vi "REV RPM to ft per s.vi"(11 "Drive Velocities (RPM)":T1) -> (3 "Drive Velocities (ft/s)":T1)   [LabVIEW 2020]
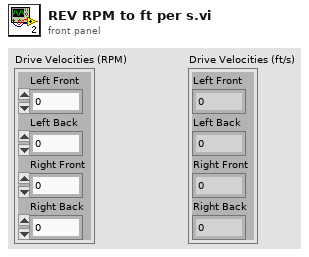
[diagram p1: front panel]
types:
  T1 = cluster{"Left Front":dbl, "Left Back":dbl, "Right Front":dbl, "Right Back":dbl}
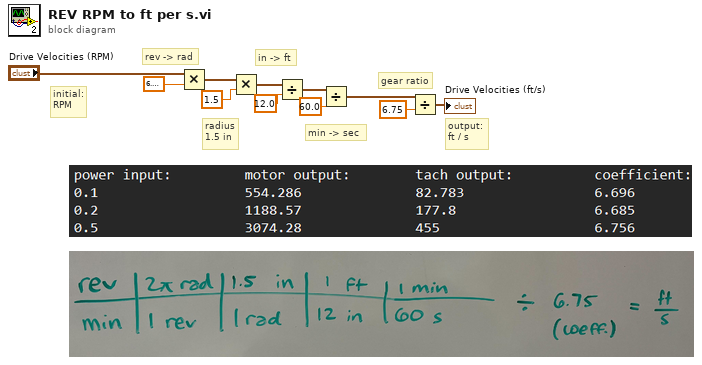
[diagram p0: block diagram]
diagram:
  # "output:\nft / s"
  # "gear ratio"
  # "min -> sec"
  # "in -> ft"
  # "initial:\nRPM"
  # "radius\n1.5 in"
  # "rev -> rad"
  n1 = Multiply(x="Drive Velocities (RPM)", y=6.283185307179586) -> (x*y=w10:T1)
  n2 = Multiply(x=w10, y=1.5) -> (x*y=w8:T1)
  n3 = Divide(x=w8, y=12.0) -> (x/y=w6:T1)
  n4 = Divide(x=w6, y=60.0) -> (x/y=w4:T1)
  n5 = Divide(x=w4, y=6.75) -> (x/y=→"Drive Velocities (ft/s)":T1)
